vi "PowX.vi"(8 "error in (no error)":errorcluster, 10 "X Value":sgl, 11 "Refnum in":T1) -> (0 "error out":errorcluster, 3 "Refnum out":T1)   [LabVIEW 2023]
uses:
  <vilib>/vision/Image Controls.llb/IMAQ Image.ctl
  HelperDLL/MP Helper.dll
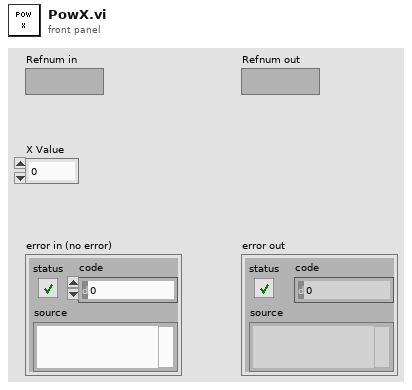
[diagram p1: front panel]
types:
  T1 = typedef "IMAQ Image.ctl" = refnum<image>
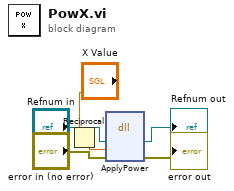
[diagram p0: block diagram]
diagram:
  n1 = Reciprocal(x="X Value") -> (1/x=w6:sgl)
  n2 = dll-call lib="C:/Users/Andrey/Desktop/xev - c leaned2/HelperDLL/MP Helper.dll" fn="ApplyPower"("Src"="Refnum in", "Power"=w6, "Err"="error in (no error)") -> ("Src"=→"Refnum out":T1, "Err"=→"error out":errorcluster)  [unwired: 5 in, 2 out]
